vi "Add_Street_Name.vi"() -> (5 "Plug in titles":string[](array[string]), 7 "Plug in values":string[](array[string]))   [LabVIEW 2020]
uses:
  Globals/Meas_global.vi
  Globals/Constants_global.vi
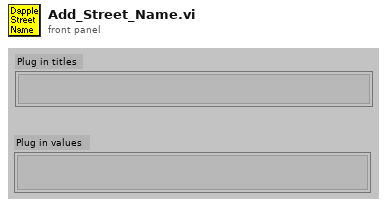
[diagram p1: front panel]
types:
  T1 = enum16{"Load setup from excel file", "Save setup to excel file"}
  T2 = enum16{"To Traverse Coordinates", "To User Coordinates"}
  T3 = typedef "Exclude_cluster.ctl" = cluster{"Sizes":T4, "Name":string, "Exclude Type":T5}
  T4 = typedef "Box_size.ctl" = cluster{"Max":dbl, "Min":dbl}[]
  T5 = typedef "Exclusion_type.ctl" = enum16{"Exclude completely", "Allow only vertical moves"}
  T6 = typedef "Post_Process.ctl" = enum16{"Take New Data", "Post Process Raw Data File"}
  T7 = typedef "Ch_description_ADAM.ctl" = cluster{"Ch Name":string, "Type":T8, "Function":T9, "Ch State":T10, "Calibration type":T11, "A":dbl, "B":dbl, "C":dbl, "D":dbl, "Comments":string, "Address":T12, "String":string, "Duty":u16}
  T8 = typedef "Module_type_ADAM.ctl" = string
  T9 = typedef "Function_ADAM.ctl" = enum16{"Analogue Input", "Digital Input", "Event counter", "Event rate", "Analogue Output", "Digital Output", "Relay Output"}
  T10 = typedef "Channel_State.ctl" = enum16{"On", "Off", "Always On", "Always Off"}
  T11 = typedef "Calib_type_ADAM.ctl" = string
  T12 = typedef "Address.ctl" = cluster{"Main":i32, "Ch.":i32, "Sub":i32, "Port Name":string}
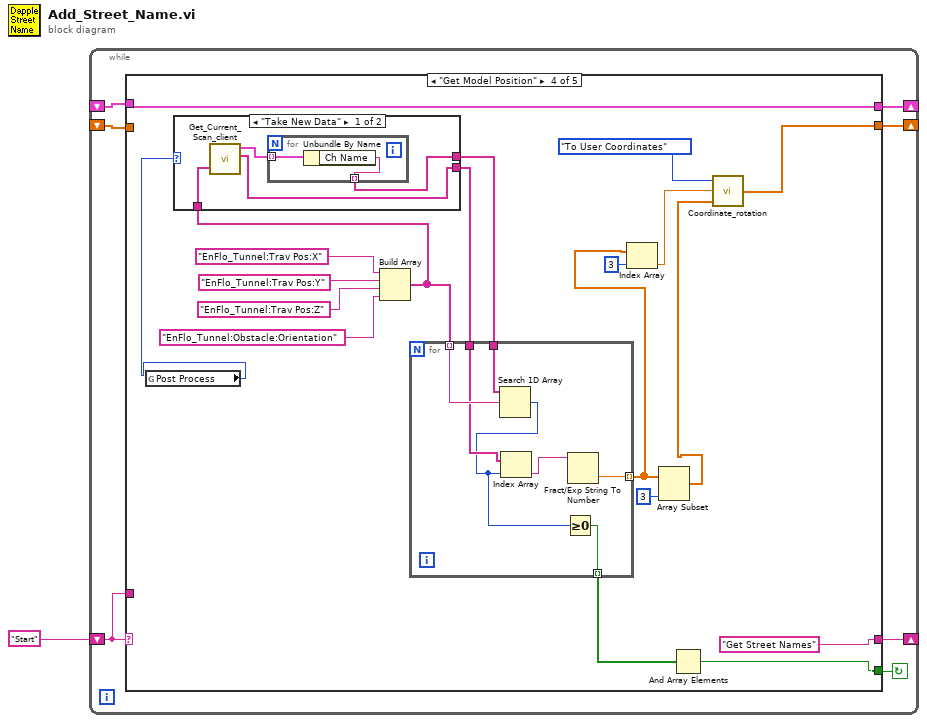
[diagram p0: block diagram]
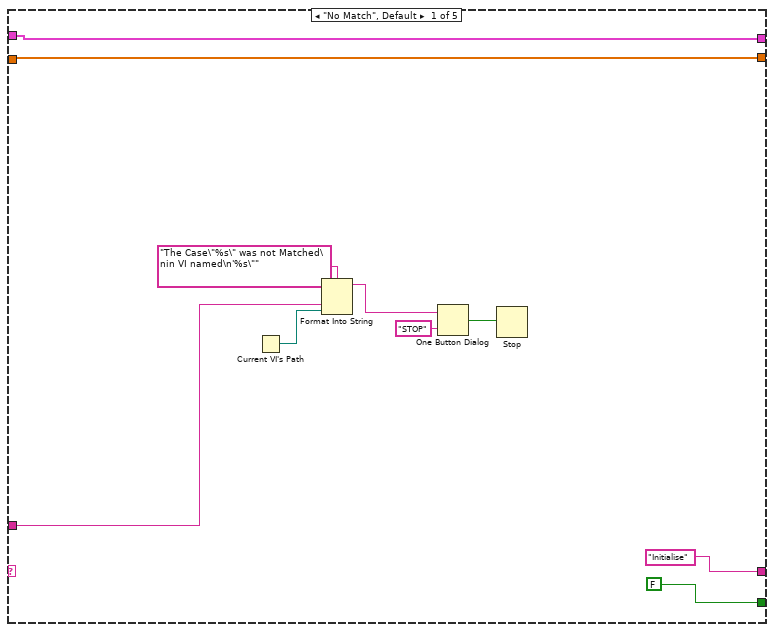
[diagram p2: hidden frame]
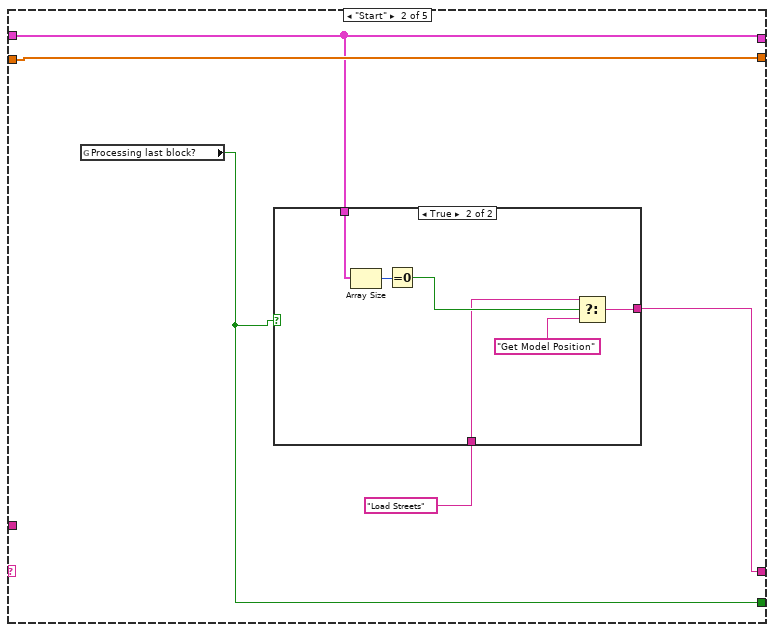
[diagram p3: hidden frame]
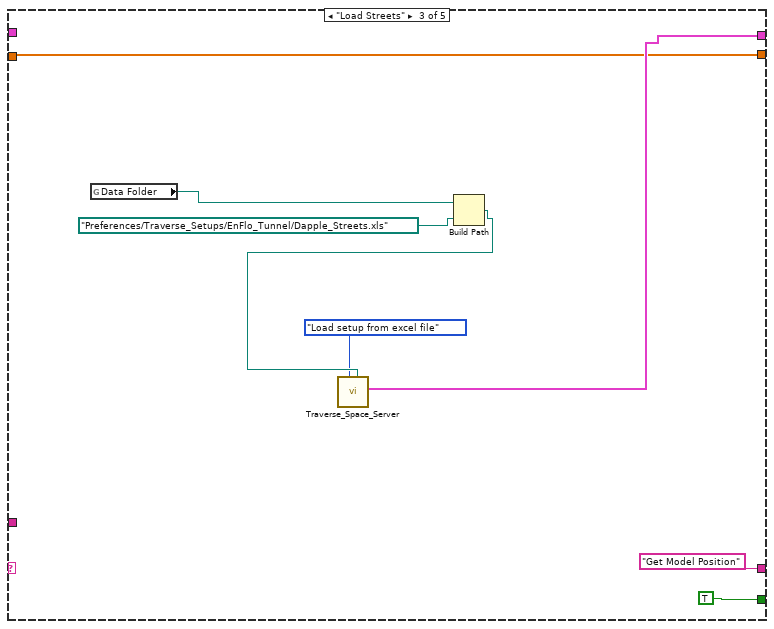
[diagram p5: hidden frame]
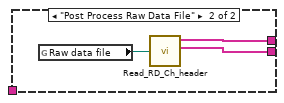
[diagram p6: hidden frame]
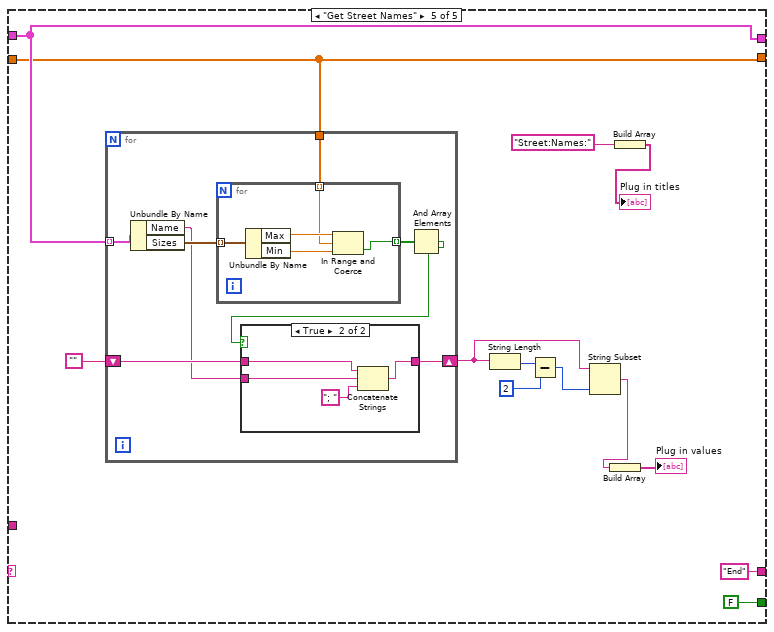
[diagram p7: hidden frame]
diagram:
  n1 = while {
    shift-left: "Start" -> [w6]
    shift-right: [w7] -> _
    shift-right: [w5] -> _
    shift-left: _ -> [w4]
    shift-right: [w3] -> _
    shift-left: _ -> [w2]
    stop <- w8 continue-if-true
    n2 = case shown="\"Get Model Position\"" w6 {
      tunnel: [FALSE w22 TRUE w46 FALSE ("Processing last block?")] -> w8
      tunnel: ["Initialise" w19 "Get Model Position" "Get Street Names" "End"] -> w7
      tunnel: w6 -> [w13 _ _ _ _]
      tunnel: [w10 w21 w32 w56 w75] -> w5
      tunnel: w4 -> [w10 w21 _ w56 w75]
      tunnel: [w9 w23 w31 w57 w74] -> w3
      tunnel: w2 -> [w9 w23 w31 _ w74]
      frame "No Match", Default {
        n3 = Current VI's Path() -> (path=w12:path)
        n4 = Format Into String(format string="The Case\"%s\" was not Matched\nin VI named\n'%s\"" ("Format String"), w13, w12) -> (resulting string=w16:string)  [unwired: 2 in, 1 out]
        n5 = One Button Dialog(message=w16, button name ("OK")="STOP") -> (true=w14:bool)
        n6 = Stop(stop? (T)=w14) -> ()
      }
      frame "Start" {
        n7 = global read "Meas_global.vi" "Processing last block?"() -> (w22:bool)
        n8 = case shown="True" w22 {
          tunnel: w21 -> [_ w30]
          tunnel: "Load Streets" -> [w24 w27]
          tunnel: [w24 w26] -> w19
          frame False {
          }
          frame True {
            n9 = Array Size(array=w30) -> (size(s)=w29:i32)
            n10 = Equal To 0?(x=w29) -> (x = 0?=w28:bool)
            n11 = Select(t=w27, s=w28, f="Get Model Position") -> (s? t:f=w26:string)
          }
        }
      }
      frame "Load Streets" {
        n12 = global read "Constants_global.vi" "Data Folder"() -> (w36:path)
        n13 = Build Path(base path=w36, name or relative path=path "Preferences/Traverse_Setups/EnFlo_Tunnel/Dapple_Streets.xls") -> (appended path=w34:path)
        n14 = call "Traverse_Space_Server.vi"("Space File"=w34, "Mode"=T1."Load setup from excel file") -> ("Exclude Array Out"=w32:T3[])  [unwired: 5 in, 3 out]
      }
      frame "Get Model Position" {
        n15 = global read "Meas_global.vi" "Post Process"() -> (w40:T6)
        n16 = Build Array("EnFlo_Tunnel:Trav Pos:X", "EnFlo_Tunnel:Trav Pos:Y", "EnFlo_Tunnel:Trav Pos:Z", "EnFlo_Tunnel:Obstacle:Orientation") -> (w39:string[])
        n17 = case shown="\"Take New Data\"" w40 {
          tunnel: [w60 w65] -> w49
          tunnel: [w59 w64] -> w48
          tunnel: w39 -> [w58 _]
          frame "Take New Data" {
            n18 = call "Get_Current_Scan_client.vi"("multipleChannels"=w58) -> ("Ch Description Array"=w61:T7[], "String values"=w59:string[])  [unwired: 2 in, 1 out]
            n19 = for {
              tunnel: w61 -> [w63] mode=indexing
              tunnel: [w62] -> w60 mode=indexing
              n20 = Unbundle By Name(w63) -> ("Ch Name"=w62:string)
            }
          }
          frame "Post Process Raw Data File" {
            n21 = global read "Meas_global.vi" "Raw data file"() -> (w66:path)
            n22 = call "Read_RD_Ch_header.vi"("Raw data file"=w66) -> ("Ch Name Out"=w65:string[], "Ch Values"=w64:string[])  [unwired: 2 out]
          }
        }
        n23 = for {
          tunnel: [w72] -> w41 mode=indexing
          tunnel: w39 -> [w71] mode=indexing
          tunnel: w49 -> [w70]
          tunnel: w48 -> [w69]
          tunnel: [w67] -> w47 mode=indexing
          n24 = Search 1D Array(1D array=w70, element=w71) -> (index of element=w68:i32)  [unwired: 1 out]
          n25 = Index Array(array=w69, index=w68) -> (element=w73:string)
          n26 = Greater Or Equal To 0?(x=w68) -> (x >= 0?=w67:bool)
          n27 = Fract/Exp String To Number(string=w73) -> (number=w72:dbl)  [unwired: 4 out]
        }
        n28 = Index Array(array=w41, index=3) -> (element=w44:dbl)
        n29 = Array Subset(array=w41, length=3) -> (w42:dbl[])  [unwired: 1 in]
        n30 = And Array Elements(Boolean array=w47) -> (logical AND=w46:bool)
        n31 = call "Coordinate_rotation.vi"("Input Position"=w42, "Coordinate rotation (deg)"=w44, "Mode"=T2."To User Coordinates") -> ("Output Position"=w57:dbl[])
      }
      frame "Get Street Names" {
        n32 = for {
          tunnel: w75 -> [w94] mode=indexing
          tunnel: w74 -> [w92]
          shift-right: [w88] -> w82
          shift-left: "" -> [w90]
          n33 = Unbundle By Name(w94) -> ("Name"=w89:string, "Sizes"=w93:T4)
          n34 = for {
            tunnel: w93 -> [w104] mode=indexing
            tunnel: w92 -> [w101] mode=indexing
            tunnel: [w100] -> w91 mode=indexing
            n35 = Unbundle By Name(w104) -> ("Max"=w103:dbl, "Min"=w102:dbl)
            n36 = In Range and Coerce(upper limit=w103, x=w101, lower limit=w102) -> (In Range?=w100:bool)  [unwired: 1 out]
          }
          n37 = And Array Elements(Boolean array=w91) -> (logical AND=w87:bool)
          n38 = case shown="True" w87 {
            tunnel: w90 -> [w95 w99]
            tunnel: w89 -> [_ w98]
            tunnel: [w95 w96] -> w88
            frame False {
            }
            frame True {
              n39 = Concatenate Strings(w99, w98, "; " ("string")) -> (w96:string)
            }
          }
        }
        n40 = String Length(string=w82) -> (length=w85:i32)
        n41 = Subtract(x=w85, y=2) -> (x-y=w83:i32)
        n42 = String Subset(string=w82, length (rest)=w83) -> (substring=w79:string)  [unwired: 1 out]
        n43 = Build Array(w79) -> (→"Plug in values":string[])
        n44 = Build Array("Street:Names:") -> (→"Plug in titles":string[])
      }
    }
  }
